vi "LU20_T_Control.vi"(0 "connection ID in":refnum<k5>, 5 "error IN":errorcluster) -> (10 "T cluster":T1, 11 "alarm cluster":T2, 14 "connection ID out":refnum<k5>, 19 "error OUT":errorcluster)   [LabVIEW 2013]
panel:
  in  "Bool cluster init":T2
  in  "init cluster":T1
  in  "Critical temp":i8=40 caption="Критическая температура"
  in  "Sens N":u8=5 caption="Количество датчиков"
  # "Колектор №1"
  # "Колектор №2"
  # "Колектор №3"
  # "Расширительный бачек"
  # "Обратка"
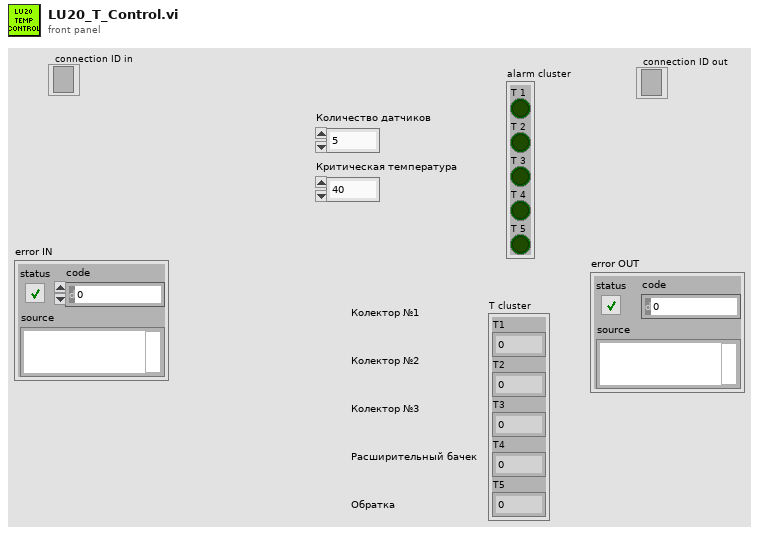
[diagram p1: front panel]
types:
  T1 = cluster{"T1":dbl, "T2":dbl, "T3":dbl, "T4":dbl, "T5":dbl}
  T2 = cluster{"T 1":bool, "T 2":bool, "T 3":bool, "T 4":bool, "T 5":bool}
  T3 = enum16{"Standard", "Buffered", "CRLF", "Immediate"}
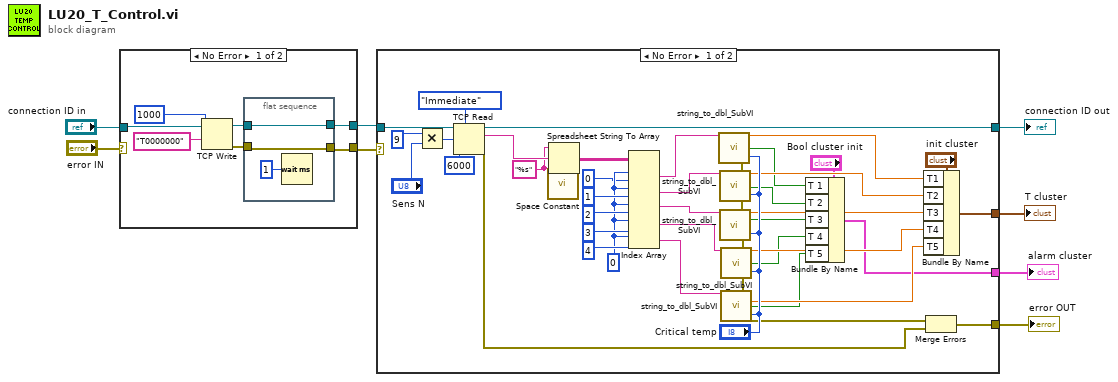
[diagram p0: block diagram]
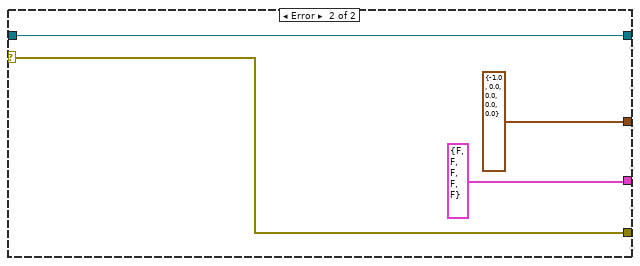
[diagram p3: hidden frame]
diagram:
  n1 = case shown="No Error" "error IN" {
    selector: "error IN" -> [_ w19]
    tunnel: "connection ID in" -> [w15 w20]
    tunnel: [w11 w20] -> w7
    tunnel: [w10 w19] -> w8
    frame No Error {
      n2 = TCP Write(connection ID=w15, data in="T0000000", 9:1000 ("timeout ms (25000)")) -> (connection ID out=w12:refnum<k5>, error out=w13:errorcluster)  [unwired: 1 in, 1 out]
      n3 = flat-sequence {
        tunnel: [w17] -> w10
        tunnel: w13 -> [w17]
        tunnel: [w16] -> w11
        tunnel: w12 -> [w16]
        frame #0 {
          n4 = Wait (ms)(milliseconds to wait=u32 1) -> ()  [unwired: 1 out]
        }
      }
    }
    frame Error {
    }
  }
  n5 = case shown="No Error" w8 {
    selector: w8 -> [_ w68]
    tunnel: w7 -> [w48 w67]
    tunnel: [w41 w68] -> w3
    tunnel: [w47 w67] -> w4
    tunnel: [w34 T1 {"T1"=-1.0, "T2"=0.0, "T3"=0.0, "T4"=0.0, "T5"=0.0} ("init cluster")] -> w1
    tunnel: [w21 T2 {"T 1"=FALSE, "T 2"=FALSE, "T 3"=FALSE, "T 4"=FALSE, "T 5"=FALSE} ("Bool cluster init")] -> w2
    frame No Error {
      w54 = 0 ("index (row)")
      w59 = "%s" ("format string")
      n6 = Multiply(x=u8 9, y="Sens N") -> (x*y=w63:u8)
      n7 = TCP Read(connection ID=w48, bytes to read=w63, 7:T3."Immediate" ("mode (standard)"), 9:6000 ("timeout ms (25000)")) -> (connection ID out=w47:refnum<k5>, data out=w60:string, error out=w24:errorcluster)  [unwired: 1 in]
      n8 = call <vilib>:"Space Constant.vi"() -> ("String"=w61:string)
      n9 = Spreadsheet String To Array(delimiter (Tab)=w61, format string=w59, spreadsheet string=w60, array type (2D Dbl)=w59) -> (array=w49:string[][])
      n10 = Index Array(array=w49, index (row) #1=w54, index (col) #1=0 ("disabled index (col)"), index (row) #2=w54, index (col) #2=1 ("disabled index (col)"), index (row) #3=w54, index (col) #3=2 ("disabled index (col)"), index (row) #4=w54, index (col) #4=3 ("disabled index (col)"), index (row) #5=w54, index (col) #5=4 ("disabled index (col)")) -> (element #1=w45:string, element #2=w44:string, element #3=w43:string, element #4=w42:string, element #5=w46:string)
      n11 = call "string_to_dbl_SubVI.vi"("input string"=w45, "max t in"="Critical temp") -> ("T"=w39:dbl, "T bool"=w32:bool, "error out"=w28:errorcluster)  [unwired: 10 in, 1 out]
      n12 = call "string_to_dbl_SubVI.vi"("input string"=w44, "error in"=w28, "max t in"="Critical temp") -> ("T"=w38:dbl, "T bool"=w31:bool, "error out"=w27:errorcluster)  [unwired: 9 in, 1 out]
      n13 = call "string_to_dbl_SubVI.vi"("input string"=w43, "error in"=w27, "max t in"="Critical temp") -> ("T"=w37:dbl, "T bool"=w30:bool, "error out"=w26:errorcluster)  [unwired: 9 in, 1 out]
      n14 = call "string_to_dbl_SubVI.vi"("input string"=w42, "error in"=w26, "max t in"="Critical temp") -> ("T"=w36:dbl, "T bool"=w29:bool, "error out"=w25:errorcluster)  [unwired: 9 in, 1 out]
      n15 = call "string_to_dbl_SubVI.vi"("input string"=w46, "error in"=w25, "max t in"="Critical temp") -> ("T"=w35:dbl, "T bool"=w22:bool, "error out"=w23:errorcluster)  [unwired: 9 in, 1 out]
      n16 = Bundle By Name(cluster="Bool cluster init", "T 1"=w32, "T 2"=w31, "T 3"=w30, "T 4"=w29, "T 5"=w22) -> (w21:T2)
      n17 = Bundle By Name(cluster="init cluster", "T1"=w39, "T2"=w38, "T3"=w37, "T4"=w36, "T5"=w35) -> (w34:T1)
      n18 = Merge Errors(w23, w24) -> (w41:errorcluster)
    }
    frame Error {
    }
  }
  "connection ID out" <- w4
  "error OUT" <- w3
  "alarm cluster" <- w2
  "T cluster" <- w1
